vi "GateControlLogic.vi"(1 "Vacuum Status":T1={"Vacuum Sensors"={"TP On"=FALSE, "IG1 On"=TRUE, "IG2On"=FALSE, "IG Vac Level"=7.206095277894153e-07, "CG1 Vac Level"=7.188197481794052e-05, "CG2 Vac Level"=7.698533430214743e-05, "IG Status"=TRUE}, "In Shot Time Window"=FALSE, "IG reading meaningful"=FALSE} {"Vacuum Sensors"."CG2 Vac Level" format="%#_2e"; "Vacuum Sensors"."CG1 Vac Level" format="%#_2e"; "Vacuum Sensors"."IG Vac Level" format="%#_2e"}, 2 "Gate Valve IG Threshold":dbl=9.9e-06 min=1e-10 max=0.0001, 3 "Gate Control":T2(ring)) -> (0 "Open Gate":bool)   [LabVIEW 2016]
uses:
  VacuumStatus.ctl
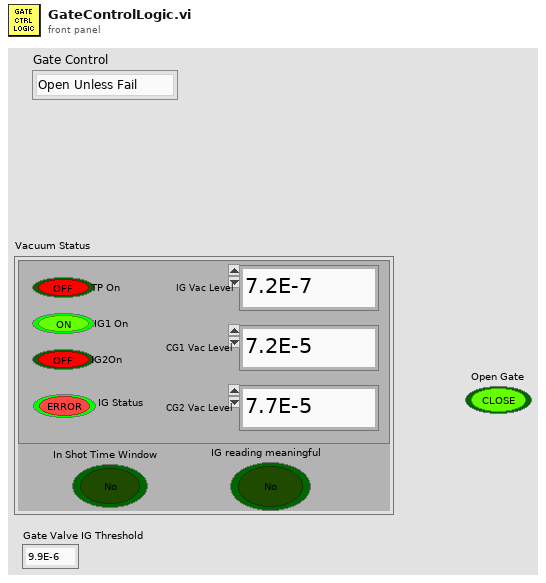
[diagram p1: front panel]
types:
  T1 = typedef "VacuumStatus.ctl" = cluster{"Vacuum Sensors":cluster{"TP On":bool, "IG1 On":bool, "IG2On":bool, "IG Vac Level":dbl, "CG1 Vac Level":dbl, "CG2 Vac Level":dbl, "IG Status":bool}, "In Shot Time Window":bool, "IG reading meaningful":bool}
  T2 = enum16{"Open Unless Fail", "Open Unless Shot", "Close"}
  T3 = cluster{"TP On":bool, "IG1 On":bool, "IG2On":bool, "IG Vac Level":dbl, "CG1 Vac Level":dbl, "CG2 Vac Level":dbl, "IG Status":bool}
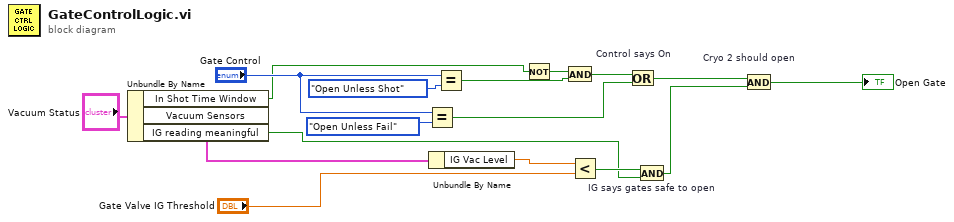
[diagram p0: block diagram]
diagram:
  n1 = Unbundle By Name("Vacuum Status") -> ("In Shot Time Window"=w2:bool, "Vacuum Sensors"=w3:T3, "IG reading meaningful"=w1:bool)
  n2 = Equal?(x="Gate Control", y=T2."Open Unless Fail") -> (x = y?=w11:bool)
  n3 = Unbundle By Name(w3) -> ("IG Vac Level"=w16:dbl)
  n4 = Equal?(x="Gate Control", y=T2."Open Unless Shot") -> (x = y?=w14:bool)
  n5 = Not(x=w2) -> (.not. x?=w13:bool)
  n6 = And(x=w13, y=w14) -> (x .and. y?=w12:bool)
  n7 = Less?(x=w16, y="Gate Valve IG Threshold") -> (x < y?=w15:bool)
  n8 = Or "Control says On"(x=w12, y=w11) -> (x .or. y?=w6:bool)
  n9 = And "IG says gates safe to open"(x=w15, y=w1) -> (x .and. y?=w7:bool)
  n10 = And "Cryo 2 should open"(x=w6, y=w7) -> (x .and. y?=→"Open Gate":bool)
